vi "BRig_dataCurrent_I_giveReward.vi"() -> (2 "output_I_giveReward":i32)   [LabVIEW 2014]
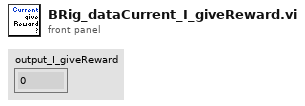
[diagram p1: front panel]
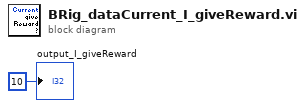
[diagram p0: block diagram]
diagram:
  "output_I_giveReward" <- 10 ("output_iBlock")
